vi "PipelineDuty.vi"(8 "error in (no error)":errorcluster, 10 "DataExchange":T1, 11 "GRMActor in":refnum<class "DataLoggerUI.lvclass">) -> (0 "error out":errorcluster, 2 "DataExchange Out":T1, 3 "GRMActor out":refnum<class "DataLoggerUI.lvclass">)   [LabVIEW 2020, in "DataLoggerUI.lvlib" / "DataLoggerUI.lvclass"]
uses:
  DataLoggerUI.lvclass
  Hardware Abstraction Layer/Component/Device/Device/DataExchange.ctl
  <vilib>/vision/Image Controls.llb/IMAQ Image.ctl
  Hardware Abstraction Layer/Component/GenericActor/GenericActor/GenericController.lvclass
  Interface/DataListener/DataListener.lvclass
panel:
  out "Source":string
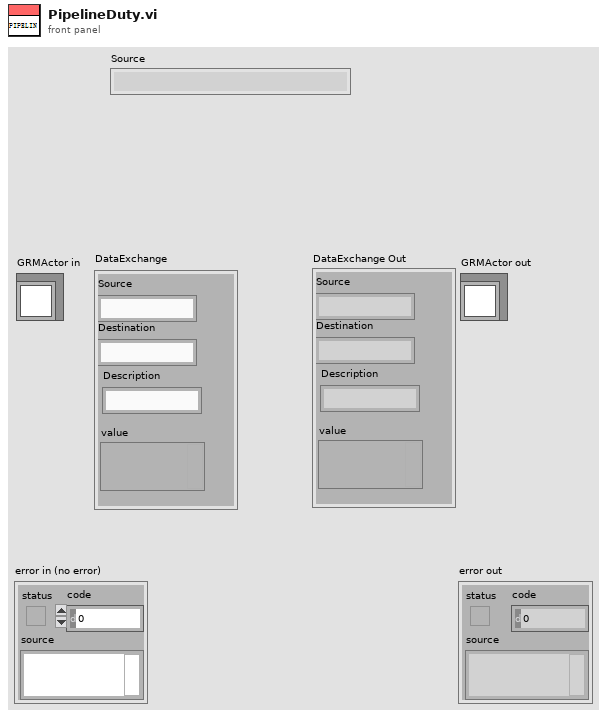
[diagram p1: front panel]
types:
  T1 = typedef "DataListener.lvclass/DataExchange.ctl" = cluster{"Source":string, "Destination":string, "Description":string, "value":variant}
  T2 = typedef "IMAQ Image.ctl" = refnum<image>
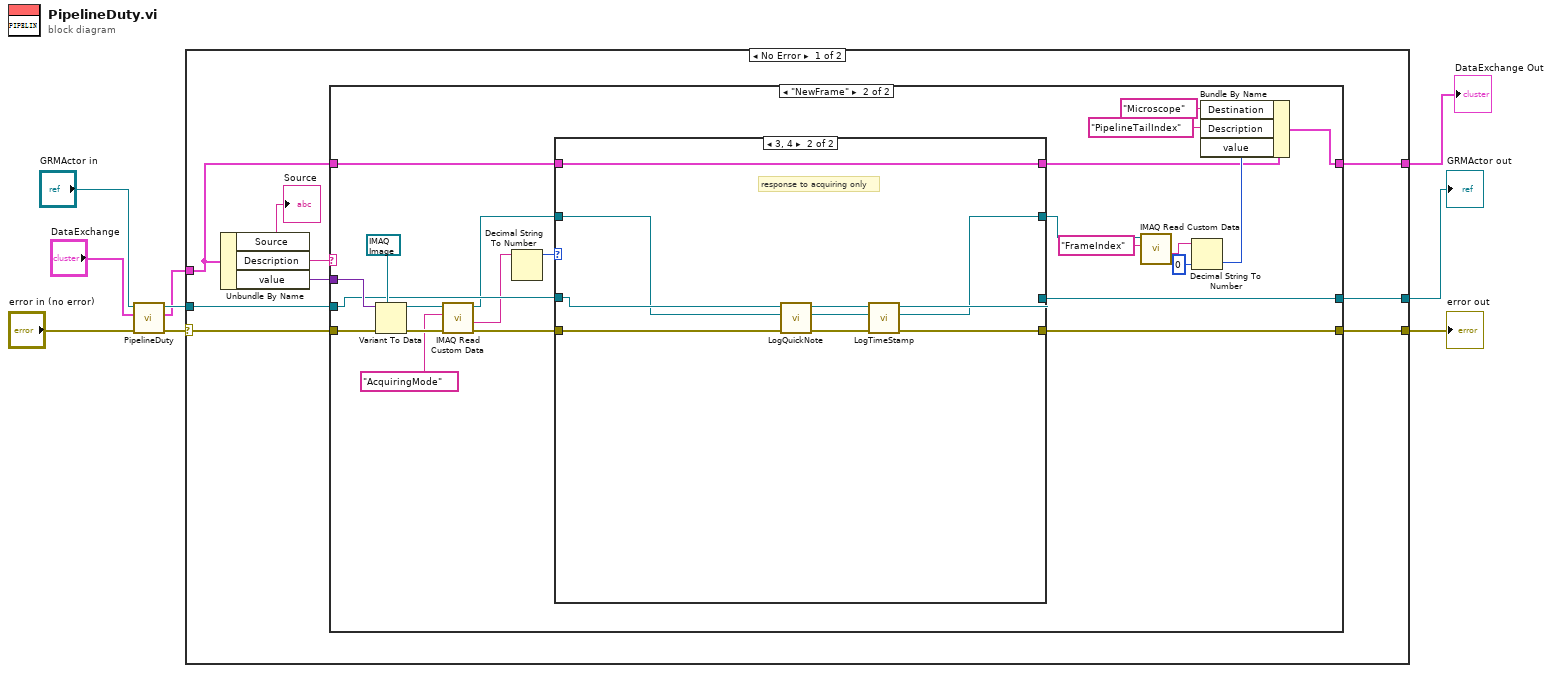
[diagram p0: block diagram]
diagram:
  n1 = call-parent "PipelineDuty.vi"("error in (no error)"="error in (no error)", "DataExchange"="DataExchange", "GRMActor in"="GRMActor in") -> ("error out"=w6:errorcluster, "DataExchange Out"=w4:T1, "GRMActor out"=w5:refnum<class "DataLoggerUI.lvclass">)  [unwired: 6 in]
  n2 = case shown="No Error" w6 {
    selector: w6 -> [w16 w61]
    tunnel: [w17 w61] -> w1
    tunnel: w5 -> [w13 w60]
    tunnel: [w18 w60] -> w2
    tunnel: w4 -> [w12 w59]
    tunnel: [w11 w59] -> w3
    frame No Error {
      n3 = Unbundle By Name(w12) -> ("Source"=→"Source":string, "Description"=w15:string, "value"=w14:variant)
      n4 = case shown="\"NewFrame\"" w15 {
        tunnel: w14 -> [_ w43]
        tunnel: [w21 w34] -> w18
        tunnel: w13 -> [w21 w35]
        tunnel: [w20 w36] -> w17
        tunnel: w16 -> [w20 w44]
        tunnel: w12 -> [w19 w40]
        tunnel: [w19 w22] -> w11
        frame Default {
        }
        frame "NewFrame" {
          n5 = Variant To Data(error in=w44, type=T2 refnum ("New Image"), Variant=w43) -> (data=w38:T2, error out=w41:errorcluster)
          n6 = call "IMAQ Read Custom Data"("error in (no error)"=w41, "Key"="AcquiringMode", "Image"=w38) -> ("error out"=w39:errorcluster, "Custom Data Out"=w32:string, "Image (duplicate)"=w33:T2)  [unwired: 6 in]
          n7 = Decimal String To Number(string=w32) -> (number=w31:i32)  [unwired: 2 in, 1 out]
          n8 = case shown="3, 4" w31 {
            tunnel: w40 -> [w48 w50]
            tunnel: [w48 w50] -> w23
            tunnel: w39 -> [w46 w58]
            tunnel: w33 -> [w45 w51]
            tunnel: [w46 w55] -> w36
            tunnel: w35 -> [w47 w56]
            tunnel: [w47 w53] -> w34
            tunnel: [w45 w49] -> w24
            frame Default {
            }
            frame 3, 4 {
              # "response to acquiring only"
              n9 = call "LogQuickNote.vi"("error in (no error)"=w58, "New Image"=w51, "GRMActor in"=w56) -> ("error out"=w57:errorcluster, "Image Out"=w52:T2, "GRMActor out"=w54:refnum<class "DataLoggerUI.lvclass">)  [unwired: 6 in]
              n10 = call "LogTimeStamp.vi"("error in (no error)"=w57, "New Image"=w52, "GRMActor in"=w54) -> ("error out"=w55:errorcluster, "Image Out"=w49:T2, "GRMActor out"=w53:refnum<class "DataLoggerUI.lvclass">)  [unwired: 6 in]
            }
          }
          n11 = call "IMAQ Read Custom Data"("Key"="FrameIndex", "Image"=w24) -> ("Custom Data Out"=w29:string)  [unwired: 7 in, 2 out]
          n12 = Decimal String To Number(string=w29, default (0L)=0 ("default (0 I32)")) -> (number=w30:i32)  [unwired: 1 in, 1 out]
          n13 = Bundle By Name(cluster=w23, "Destination"="Microscope", "Description"="PipelineTailIndex", "value"=w30) -> (w22:T1)
        }
      }
    }
    frame Error {
    }
  }
  "error out" <- w1
  "GRMActor out" <- w2
  "DataExchange Out" <- w3
